vi "Read UID.vi"(8 "error in (no error)":errorcluster, 11 "Control in":refnum<class "GObject.lvclass">) -> (0 "error out":errorcluster, 2 "UID":i32, 3 "Control out":refnum<class "GObject.lvclass">)   [LabVIEW 2013, in "SET Project Data.lvlib" / "GObject.lvclass"]
uses:
  GObject.lvclass
  GObject.lvclass/GObject.ctl
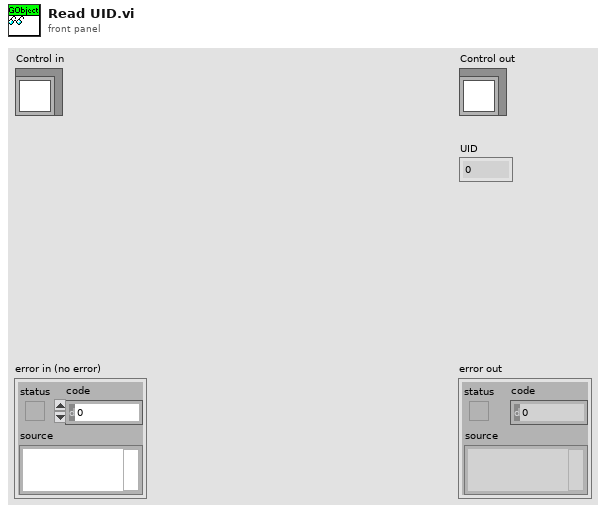
[diagram p1: front panel]
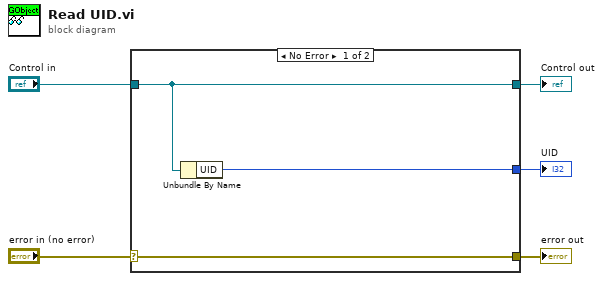
[diagram p0: block diagram]
diagram:
  n1 = case shown="No Error" "error in (no error)" {
    selector: "error in (no error)" -> [w8 w9]
    tunnel: [w8 w9] -> w4
    tunnel: [w7 w10] -> w2
    tunnel: "Control in" -> [w7 w10]
    tunnel: [w6 _] -> w1
    frame No Error {
      n2 = Unbundle By Name(w7) -> ("UID"=w6:i32)
    }
    frame Error {
    }
  }
  "error out" <- w4
  "Control out" <- w2
  "UID" <- w1
